vi "Data logger.vi"   [LabVIEW 2019]
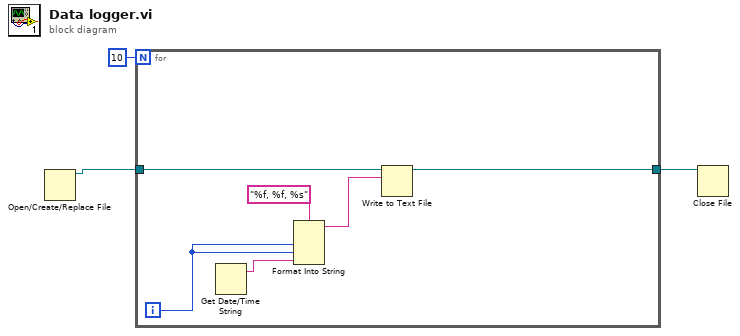
[diagram p0: block diagram]
diagram:
  n1 = Open/Create/Replace File() -> (refnum out=w2:refnum<file>)  [unwired: 6 in, 2 out]
  n2 = for {
    N: 10 -> [_]
    tunnel: w2 -> [w9]
    tunnel: [w8] -> w1
    i -> [w6]
    n3 = Get Date/Time String() -> (date string=w5:string)  [unwired: 3 in, 1 out]
    n4 = Format Into String(format string="%f, %f, %s", w6, w6, w5) -> (resulting string=w4:string)  [unwired: 2 in, 1 out]
    n5 = Write to Text File(file (use dialog)=w9, text=w4) -> (refnum out=w8:refnum<file>)  [unwired: 2 in, 2 out]
  }
  n6 = Close File(refnum=w1) -> ()  [unwired: 1 in, 2 out]
